vi "StepActionPassOrFail.vi"(5 "Result":string, 7 "Expected":string) -> (8 "Results":T1)   [LabVIEW 2023]
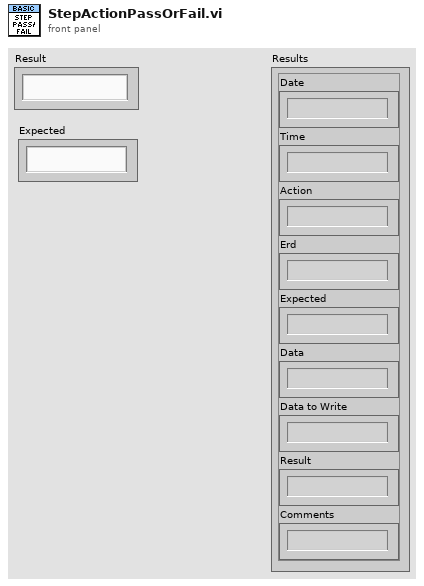
[diagram p1: front panel]
types:
  T1 = cluster{"Date":string, "Time":string, "Action":string, "Erd":string, "Expected":string, "Data":string, "Data to Write":string, "Result":string, "Comments":string}
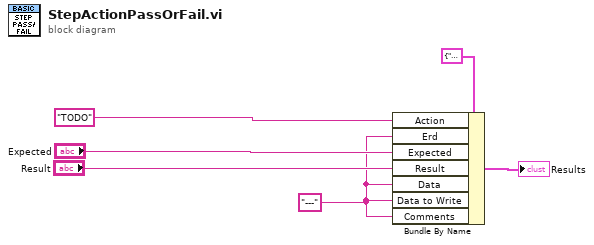
[diagram p0: block diagram]
diagram:
  w1 = "---" ("Data to Write")
  n1 = Bundle By Name(cluster=T1 {"Date"="", "Time"="", "Action"="", "Erd"="", "Expected"="", "Data"="", "Data to Write"="", "Result"="", "Comments"=""}, "Action"="TODO", "Erd"=w1, "Expected"="Expected", "Result"="Result", "Data"=w1, "Data to Write"=w1, "Comments"=w1) -> (→"Results":T1)
